vi "Reset.vi"(8 "error in (no error)":errorcluster, 11 "NhRegenGridSim in":refnum<class "NHRGridSim.lvclass">) -> (0 "error out":errorcluster, 3 "NhRegenGridSim out":refnum<class "NHRGridSim.lvclass">)   [LabVIEW 2018, in "AcPwrPlugins.lvlib" / "NHRGridSim.lvclass"]
doc: "This VI resets the instrument to <B>original power on configuration</B>. Does not clear Enable register for Standard Summary Status or Standard Event Registers. Does not clear the output queue. Does not clear the power-on-status-clear flag."
uses:
  NHRGridSim.lvclass
  <instrlib>/NH Research 9400 Series/NH Research 9400 Series.lvlib
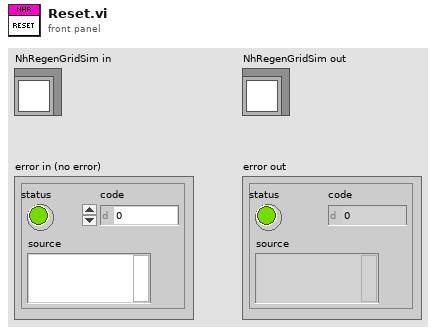
[diagram p1: front panel]
types:
  T1 = typedef "AcPwrPlugins.lvlib/NHRGridSim.lvclass/DeviceSettings.ctl" = cluster{"SlewRates":cluster{"Islew":dbl, "Vslew":dbl, "Pslew":dbl, "FreqSlew":dbl, "AngleABSlew":dbl, "AngleACSlew":dbl}, "Phases":cluster{"Pout (W)":dbl, "Iout (A)":dbl, "PhaseAngle":dbl, "Vout (V)":dbl, "Phase Name":string}[], "Measurement":cluster{"ApertureLength (s)":dbl, "NumberOfSamples":u32}, "Ranges":cluster{"Irange (A)":dbl, "Vrange (V)":dbl}, "Mode":enum8{"One 3-Phase AC", "One AC", "One DC", "Three AC", "Three DC", "One 2-Phase AC and One AC", "One 2-Phase AC and One DC", "Two AC", "One AC and One DC", "Two AC and One DC", "One AC and Two DC", "One DC and One AC", "Two DC"}, "PowerMax":u16, "TransformerRatio":dbl, "Waveshape":dbl[], "Handle":string, "FreqOut (Hz)":dbl, "Connected":bool, "Safety Limits":cluster{"Minimum Voltage (V)":dbl, "Minimum Voltage Time (s)":dbl, "Maximum Voltage (V)":dbl, "Maximum Voltage Time (s)":dbl, "Maximum Source Amps (A)":dbl, "Maximum Source Amps Time (s)":dbl, "Maximum Sink Amps (A)":dbl, "Maximum Sink Amps Time (s)":dbl, "Maximum Source Power (W)":dbl, "Maximum Source Power Time (s)":dbl, "Maximum Sink Power (W)":dbl, "Maximum Sink Power Time (s)":dbl, "Peak Voltage (V)":dbl, "Peak Voltage Enable":bool, "Peak Amps (A)":dbl, "Peak Amps Enable":bool}, "btnIdQuery":bool, "btnReset":bool, "Initialize Timeout (10000 ms)":u32}[]
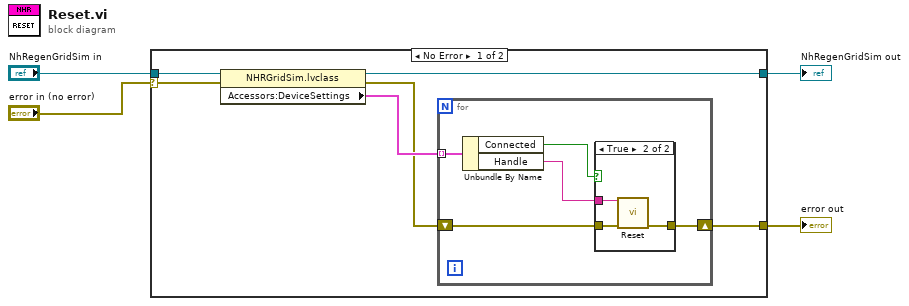
[diagram p0: block diagram]
diagram:
  n1 = case shown="No Error" "error in (no error)" {
    selector: "error in (no error)" -> [w7 w20]
    tunnel: "NhRegenGridSim in" -> [w8 w21]
    tunnel: [w6 w21] -> w2
    tunnel: [w5 w20] -> w1
    frame No Error {
      n2 = property class="NHRGridSim.lvclass"(reference=w8, error in=w7) -> (reference out=w6:refnum<class "NHRGridSim.lvclass">, error out=w9:errorcluster, "Accessors:DeviceSettings"=w10:T1)
      n3 = for {
        tunnel: w10 -> [w15] mode=indexing
        shift-right: [w12] -> w5
        shift-left: w9 -> [w13]
        n4 = Unbundle By Name(w15) -> ("Connected"=w11:bool, "Handle"=w14:string)
        n5 = case shown="True" w11 {
          tunnel: w14 -> [_ w19]
          tunnel: w13 -> [w16 w18]
          tunnel: [w16 w17] -> w12
          frame False {
          }
          frame True {
            n6 = call <instrlib>:"Reset.vi"("VISA resource name"=w19, "error in (no error)"=w18) -> ("error out"=w17:errorcluster)  [unwired: 12 in, 1 out]
          }
        }
      }
    }
    frame Error {
    }
  }
  "error out" <- w1
  "NhRegenGridSim out" <- w2
